vi "FringeTracker-HandPaddle.vi"() -> ()   [LabVIEW 2009]
uses:
  Instruments/RTC/Api/TelemetryServer/TelemetryServer_Global.vi
panel:
  out "DLPosition History":dbl[unit](graph)
  out "DLPosition":dbl format="%.6g"
  in  "Step Sixe":dbl[unit](slide) scale format="%#.1f"
  in  "stop":bool
  in  ">":bool
  in  "<":bool
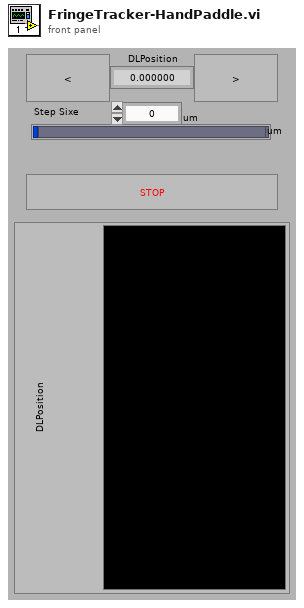
[diagram p1: front panel]
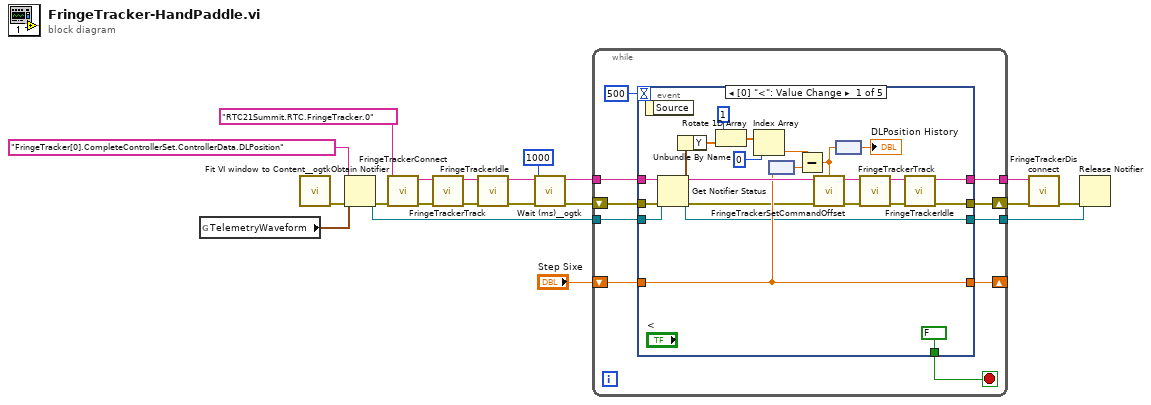
[diagram p0: block diagram]
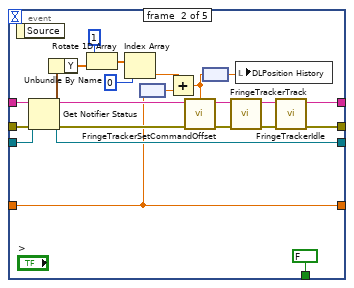
[diagram p2: hidden frame]
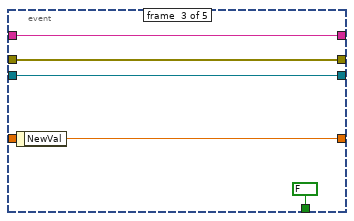
[diagram p3: hidden frame]
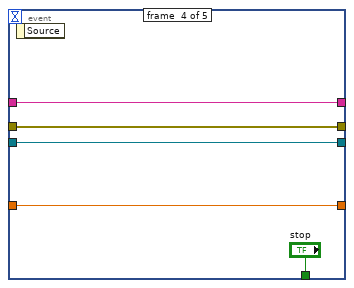
[diagram p4: hidden frame]
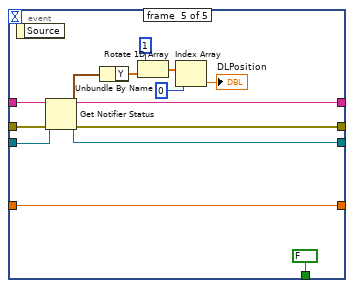
[diagram p5: hidden frame]
diagram:
  n1 = global read "TelemetryServer_Global.vi" "TelemetryWaveform"() -> (w16:waveform(dbl))
  n2 = call <userlib>:"Fit VI window to Content__ogtk.vi"() -> ("error out"=w4:errorcluster)  [unwired: 3 in, 4 out]
  n3 = Obtain Notifier(name (unnamed)="FringeTracker[0].CompleteControllerSet.ControllerData.DLPosition" ("nom (aucun)"), notification data type=w16, error in (no error)=w4) -> (notifier out=w14:refnum<notifier>, error out=w15:errorcluster)  [unwired: 1 in, 1 out]
  n4 = call "FringeTrackerConnect.vi"("FringeTracker Name"="RTC21Summit.RTC.FringeTracker.0", "error in (no error)"=w15) -> ("FringeTracker Name out"=w9:string, "error out"=w6:errorcluster)  [unwired: 6 out]
  n5 = call "FringeTrackerTrack.vi"("error in (no error)"=w6, "FringeTracker Name"=w9) -> ("error out"=w5:errorcluster, "FringeTracker Name out"=w8:string)  [unwired: 6 out]
  n6 = call "FringeTrackerIdle.vi"("error in (no error)"=w5, "FringeTracker Name"=w8) -> ("error out"=w3:errorcluster, "FringeTracker Name out"=w7:string)  [unwired: 6 out]
  n7 = call <userlib>:"Wait (ms)__ogtk.vi"("error in (no error)"=w3, "milliseconds to wait"=u32 1000) -> ("error out"=w2:errorcluster)  [unwired: 1 in, 8 out]
  n8 = while {
    shift-right: [w24] -> w13
    shift-left: w2 -> [w29]
    shift-right: [w27] -> _
    shift-left: "Step Sixe" -> [w28]
    tunnel: w7 -> [w26]
    tunnel: w14 -> [w25]
    tunnel: [w23] -> w12
    tunnel: [w22] -> w10
    stop <- w21 stop-if-true
    n9 = event shown="[0] \"<\": Value Change" {
      selector: _ -> [_ _ _ _ _]
      dyn-events: _ -> [_ _ _ _ _]
      timeout: 500 -> [_ _ _ _ _]
      tunnel: w29 -> [w36 w71 w76 w80 w89]
      tunnel: w28 -> [w49 w67 _ w82 w91]
      tunnel: [w49 w67 w78 w82 w91] -> w27
      tunnel: w26 -> [w51 w69 w75 w79 w93]
      tunnel: w25 -> [w35 w70 w77 w81 w96]
      tunnel: [w33 w68 w77 w81 w95] -> w22
      tunnel: [w43 w62 w76 w80 w94] -> w24
      tunnel: [w44 w61 w75 w79 w93] -> w23
      tunnel: [FALSE ("stop") FALSE ("stop") FALSE ("stop") "stop" FALSE ("stop")] -> w21
      event #0 {
        n10 = event-data() -> ()  [unwired: 2 out]
        n11 = Get Notifier Status(notifier=w35, error in (no error)=w36) -> (notifier out=w33:refnum<notifier>, current notification=w32:waveform(dbl), error out=w34:errorcluster)  [unwired: 2 out]
        n12 = Unbundle By Name(w32) -> ("Y"=w41:dbl[])
        n13 = Rotate 1D Array(1:w41, 2:1 ("n")) -> (0:w39:dbl[])
        n14 = Index Array(array=w39, index=0 ("indice")) -> (element=w37:dbl)
        n15 = node(w49) -> (w50:dbl)
        n16 = Subtract(x=w37, y=w50) -> (x-y=w31:dbl)
        n17 = call "FringeTrackerSetCommandOffset.vi"("offset"=w31, "FringeTracker Name"=w51, "error in (no error)"=w34) -> ("FringeTracker Name out"=w47:string, "error out"=w48:errorcluster)  [unwired: 5 out]
        n18 = node(w31) -> (→"DLPosition History":dbl[unit])
        n19 = call "FringeTrackerTrack.vi"("error in (no error)"=w48, "FringeTracker Name"=w47) -> ("error out"=w46:errorcluster, "FringeTracker Name out"=w45:string)  [unwired: 6 out]
        n20 = call "FringeTrackerIdle.vi"("error in (no error)"=w46, "FringeTracker Name"=w45) -> ("error out"=w43:errorcluster, "FringeTracker Name out"=w44:string)  [unwired: 6 out]
      }
      event #1 {
        n21 = event-data() -> ()  [unwired: 2 out]
        n22 = Get Notifier Status(notifier=w70, error in (no error)=w71) -> (notifier out=w68:refnum<notifier>, current notification=w55:waveform(dbl), error out=w73:errorcluster)  [unwired: 2 out]
        n23 = Unbundle By Name(w55) -> ("Y"=w59:dbl[])
        n24 = Rotate 1D Array(1:w59, 2:1 ("n")) -> (0:w57:dbl[])
        n25 = Index Array(array=w57, index=0 ("indice")) -> (element=w54:dbl)
        n26 = node(w67) -> (w72:dbl)
        n27 = Add(x=w54, y=w72) -> (x+y=w53:dbl)
        n28 = call "FringeTrackerSetCommandOffset.vi"("offset"=w53, "FringeTracker Name"=w69, "error in (no error)"=w73) -> ("FringeTracker Name out"=w64:string, "error out"=w65:errorcluster)  [unwired: 5 out]
        n29 = node(w53) -> (w52:dbl[unit])
        n30 = call "FringeTrackerTrack.vi"("error in (no error)"=w65, "FringeTracker Name"=w64) -> ("error out"=w63:errorcluster, "FringeTracker Name out"=w66:string)  [unwired: 6 out]
        n31 = local write "DLPosition History"(w52) -> ()
        n32 = call "FringeTrackerIdle.vi"("error in (no error)"=w63, "FringeTracker Name"=w66) -> ("error out"=w62:errorcluster, "FringeTracker Name out"=w61:string)  [unwired: 6 out]
      }
      event #2 {
        n33 = event-data() -> ("NewVal"=w78:dbl[unit])  [unwired: 1 out]
      }
      event #3 {
        n34 = event-data() -> ()  [unwired: 2 out]
      }
      event #4 {
        n35 = event-data() -> ()  [unwired: 2 out]
        n36 = Get Notifier Status(notifier=w96, error in (no error)=w89) -> (notifier out=w95:refnum<notifier>, current notification=w90:waveform(dbl), error out=w94:errorcluster)  [unwired: 2 out]
        n37 = Unbundle By Name(w90) -> ("Y"=w88:dbl[])
        n38 = Rotate 1D Array(1:w88, 2:1 ("n")) -> (0:w86:dbl[])
        n39 = Index Array(array=w86, index=0 ("indice")) -> (element=→"DLPosition":dbl)
      }
    }
  }
  n40 = call "FringeTrackerDisconnect.vi"("FringeTracker Name"=w12, "error in (no error)"=w13) -> ("error out"=w11:errorcluster)  [unwired: 7 out]
  n41 = Release Notifier(notifier=w10, error in (no error)=w11) -> ()  [unwired: 4 out]
